vi "GetPolyInstanceInfo.vi"(8 "error in (no error)":errorcluster, 11 "Poly VI Path":path) -> (0 "error out":errorcluster, 2 "InstanceInfo":T1(array[cluster]), 3 "VI Name":string)   [LabVIEW 2020]
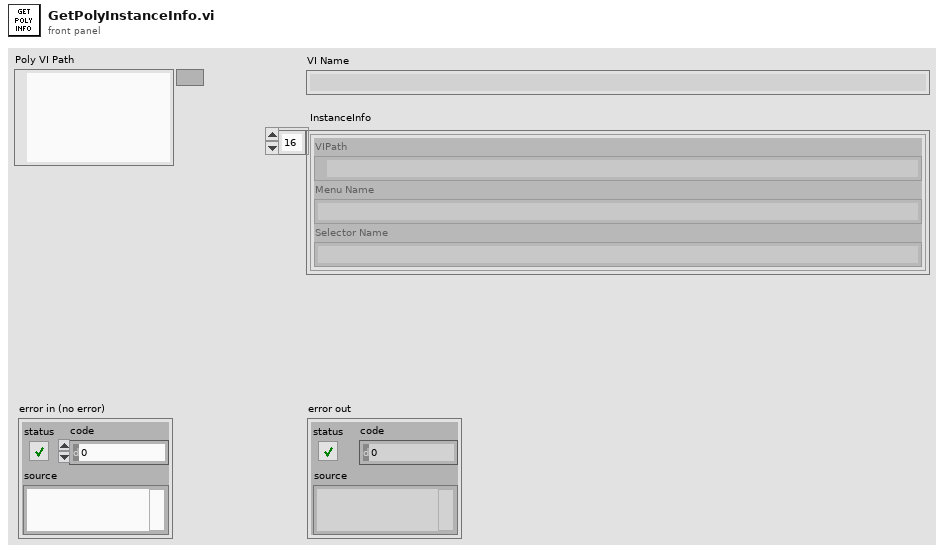
[diagram p1: front panel]
types:
  T1 = cluster{"VIPath":path, "Menu Name":string, "Selector Name":string}[]
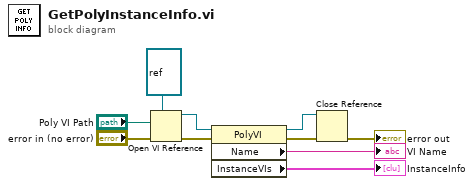
[diagram p0: block diagram]
diagram:
  n1 = Open VI Reference(type specifier VI Refnum (for type only)=refnum<vi> refnum, vi path="Poly VI Path", error in (no error)="error in (no error)") -> (vi reference=w8:refnum<vi>, error out=w7:errorcluster)  [unwired: 3 in]
  n2 = property class="PolyVI"(reference=w8, error in=w7) -> (reference out=w3:refnum<vi>, error out=w4:errorcluster, "Name"=→"VI Name":string, "InstanceVIs"=→"InstanceInfo":T1)
  n3 = Close Reference(reference=w3, error in (no error)=w4) -> (error out=→"error out":errorcluster)
